vi "meTEC_Decompose Serial Message.vi"(8 "error in (no error)":errorcluster, 11 "Serial Message IN":string) -> (0 "error out":errorcluster, 2 "Payload (e.g. Temperature)":dbl format="%#.3f")   [LabVIEW 2010]
panel:
  out "Payload (e.g. Temperature)":string
  out "CRC (Calculated)":string
  out "CRC (from TEC)":string
  out "Sequence Number":string
  out "Address":string
  out "Control":string
  # "--- Outputs ---"
  # "--- Inputs ---"
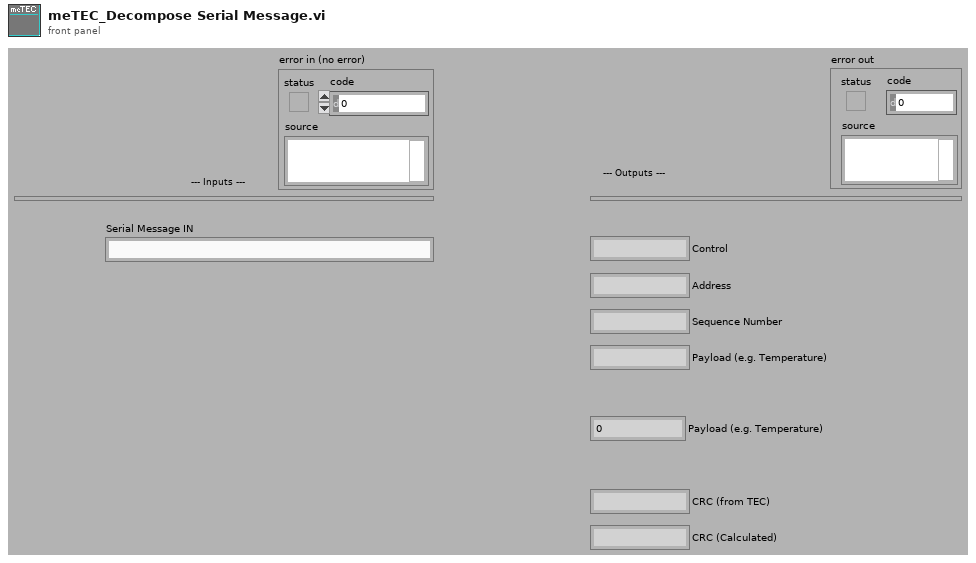
[diagram p1: front panel]
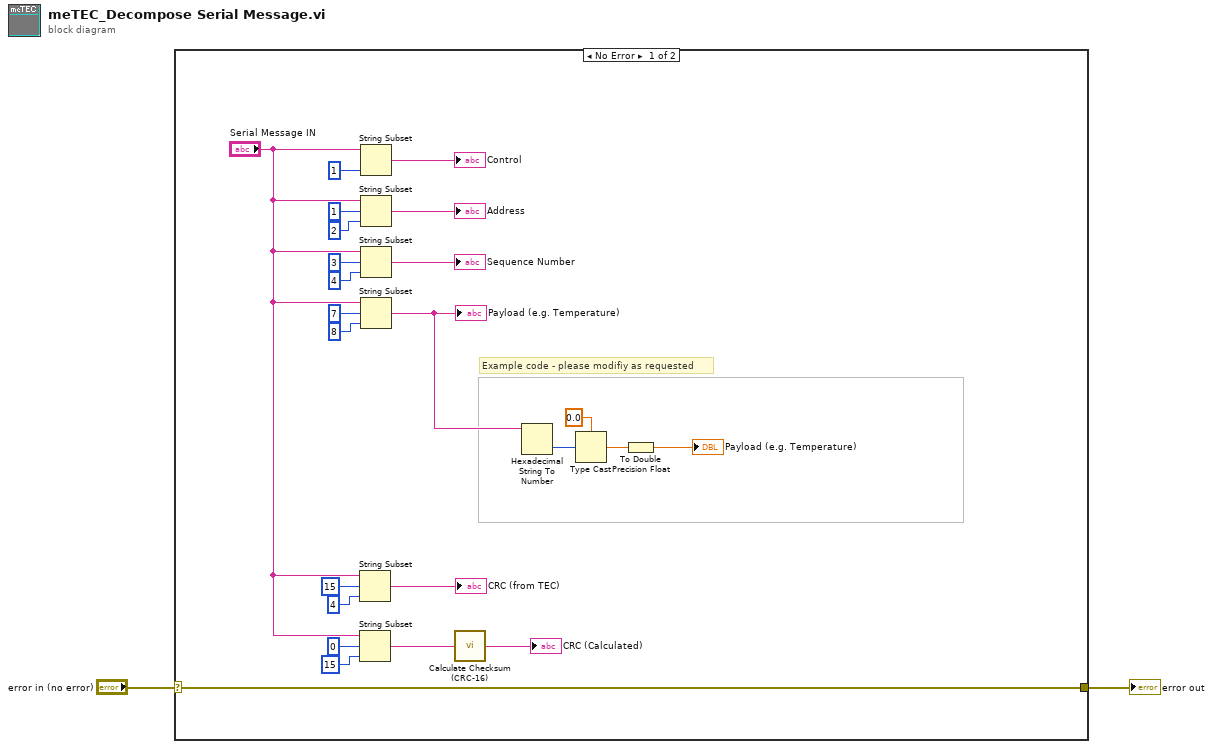
[diagram p0: block diagram]
diagram:
  n1 = case shown="No Error" "error in (no error)" {
    selector: "error in (no error)" -> [w3 w27]
    tunnel: [w3 w27] -> w1
    frame No Error {
      # "Example code - please modifiy as requested"
      n2 = String Subset(string="Serial Message IN", offset (0)=15, length (rest)=4 ("length (rest)")) -> (substring=→"CRC (from TEC)":string)
      n3 = String Subset(string="Serial Message IN", offset (0)=0, length (rest)=15 ("length (rest)")) -> (substring=w11:string)
      n4 = String Subset(string="Serial Message IN", length (rest)=1 ("length (rest)")) -> (substring=→"Control":string)  [unwired: 1 in]
      n5 = String Subset(string="Serial Message IN", offset (0)=1, length (rest)=2 ("length (rest)")) -> (substring=→"Address":string)
      n6 = String Subset(string="Serial Message IN", offset (0)=3, length (rest)=4 ("length (rest)")) -> (substring=→"Sequence Number":string)
      n7 = String Subset(string="Serial Message IN", offset (0)=7, length (rest)=8 ("length (rest)")) -> (substring=w5:string)
      "Payload (e.g. Temperature)" <- w5
      n8 = call "Calculate Checksum (CRC-16).vi"("Message"=w11) -> ("CRC [String]"=→"CRC (Calculated)":string)  [unwired: 1 in]
      n9 = Hexadecimal String To Number(string=w5) -> (number=w4:u32)  [unwired: 2 in, 1 out]
      n10 = Type Cast(type=sgl 0.0, x=w4) -> (*(type *) &x=w7:sgl)
      n11 = To Double Precision Float(number=w7) -> (double precision float=→"Payload (e.g. Temperature)":dbl)
    }
    frame Error {
    }
  }
  "error out" <- w1
